vi "NI 9265 DOUBLE TASK.vi"(8 "error in":errorcluster, 11 "MODULE NAME":string="CDR_AO1") -> (0 "error out":errorcluster, 3 "task out":refnum<k21>)   [LabVIEW 2019]
uses:
  <vilib>/DAQmx/create/channels.llb/DAQmx Create Channel (AO-Current-Basic).vi
  <resource>/objmgr/daqmx.rc
panel:
  out "error out 2":errorcluster
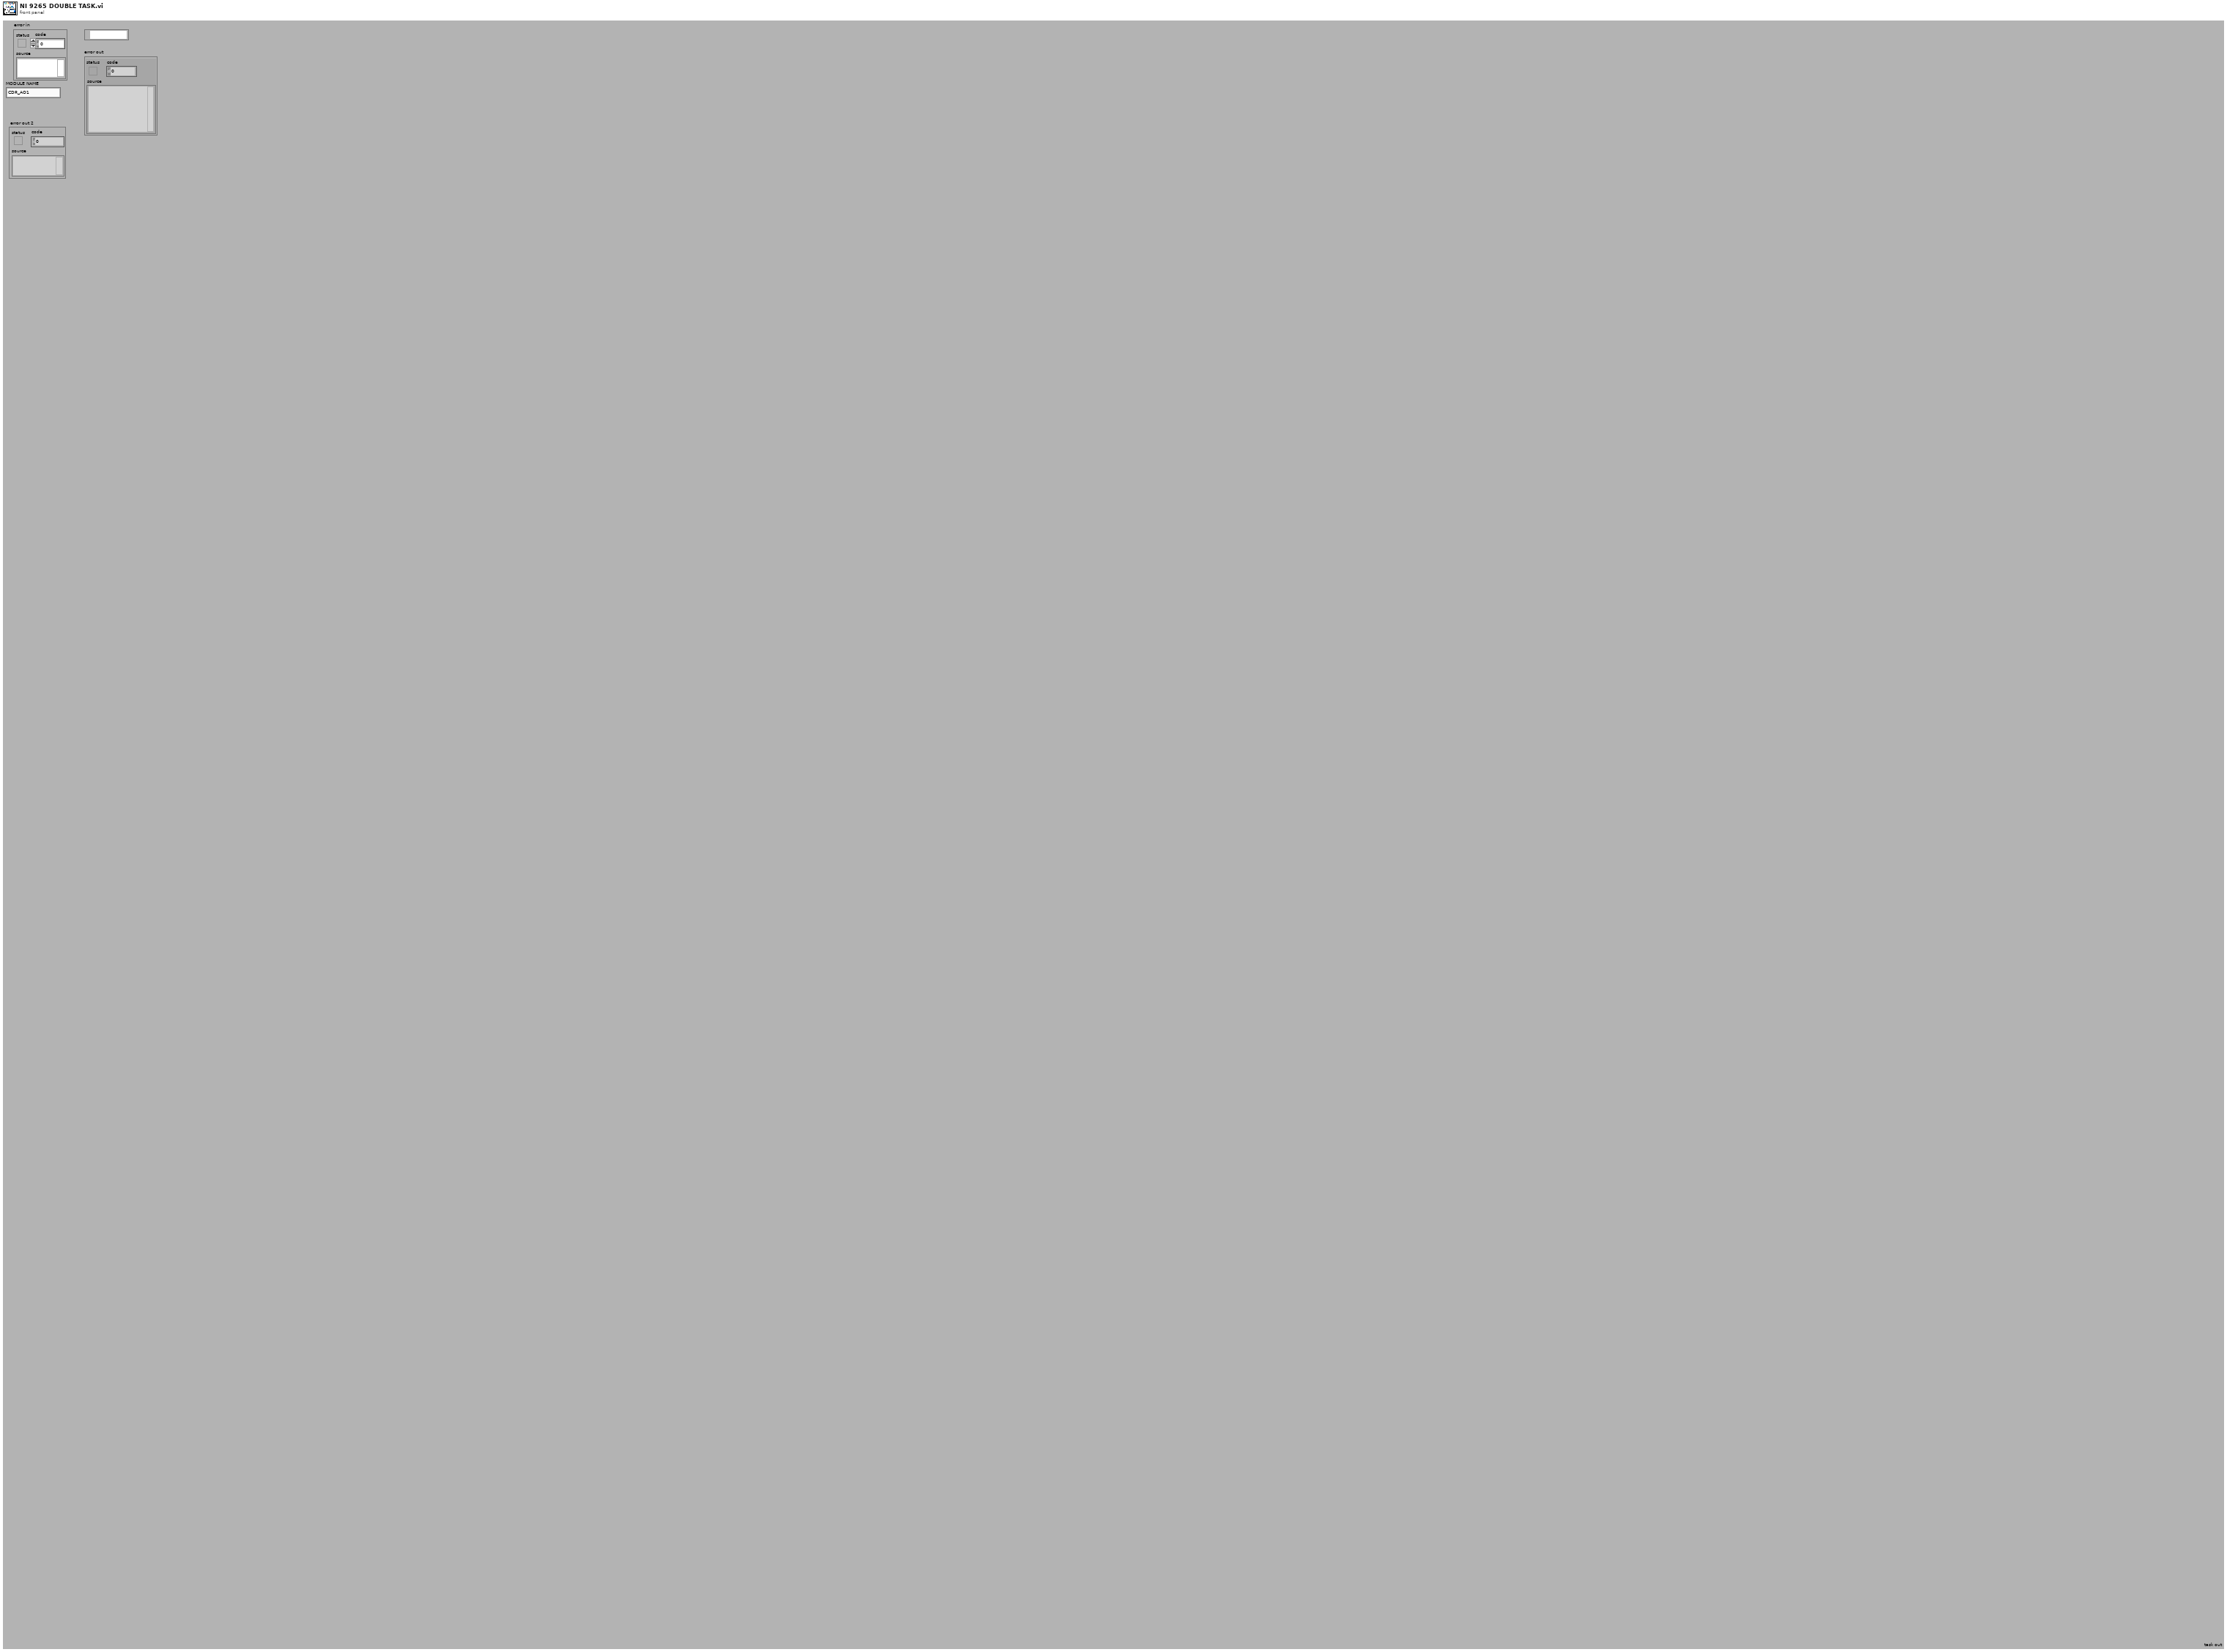
[diagram p1: front panel]
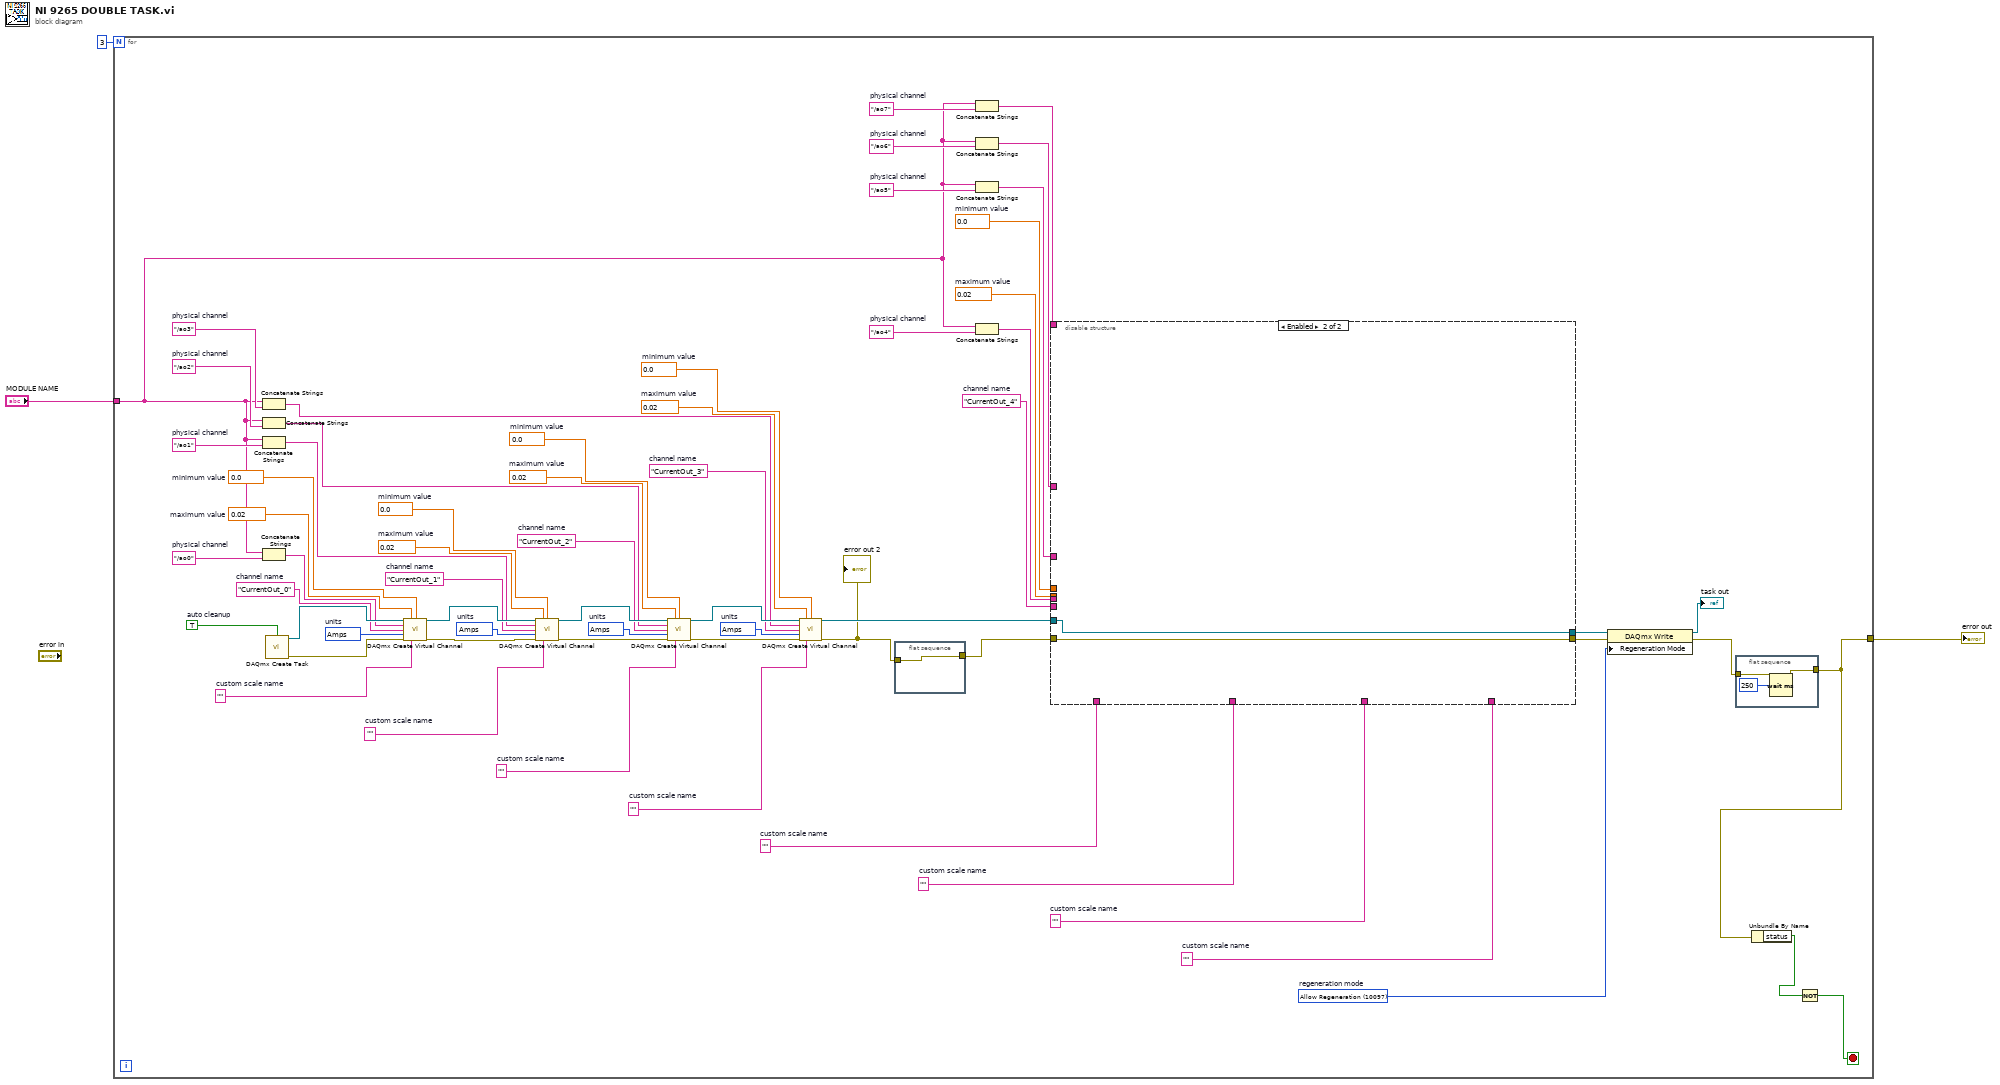
[diagram p0: block diagram]
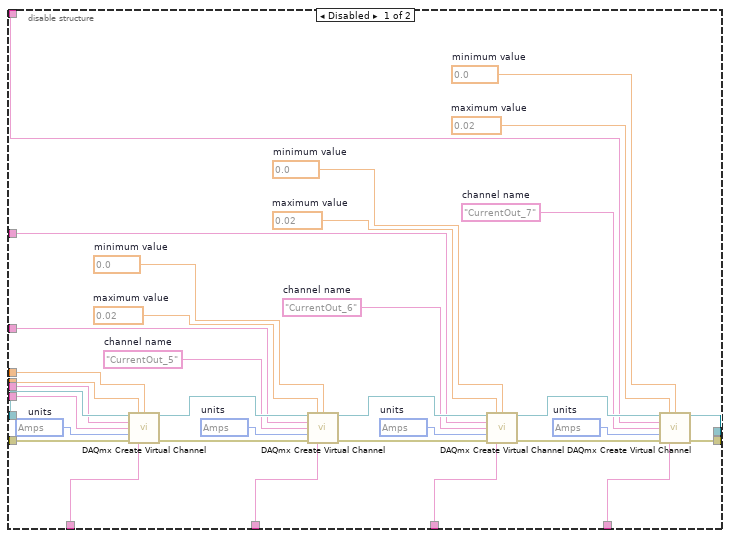
[diagram p2: hidden frame]
diagram:
  n1 = for {
    N: 3 -> [_]
    tunnel: "MODULE NAME" -> [w5]
    tunnel: [w8] -> w1
    stop <- w6 stop-if-true
    w13 = "/ao7"  # physical channel
    w15 = "/ao6"  # physical channel
    w17 = "/ao5"  # physical channel
    w20 = "CurrentOut_4"  # channel name
    w21 = 0.0  # minimum value
    w22 = 0.02  # maximum value
    w19 = "/ao4"  # physical channel
    w34 = 10097 items=["Allow Regeneration"=10097, "Do Not Allow Regeneration"=10158]  # regeneration mode
    w35 = ""  # custom scale name
    w36 = ""  # custom scale name
    w37 = ""  # custom scale name
    w38 = ""  # custom scale name
    w40 = 10342 items=["Amps"=10342, "From Custom Scale"=10065]  # units
    w41 = "CurrentOut_3"  # channel name
    w42 = ""  # custom scale name
    w43 = 0.0  # minimum value
    w44 = 0.02  # maximum value
    w25 = "/ao3"  # physical channel
    w46 = 10342 items=["Amps"=10342, "From Custom Scale"=10065]  # units
    w47 = "CurrentOut_2"  # channel name
    w49 = ""  # custom scale name
    w50 = 0.0  # minimum value
    w51 = 0.02  # maximum value
    w27 = "/ao2"  # physical channel
    w53 = 10342 items=["Amps"=10342, "From Custom Scale"=10065]  # units
    w54 = "CurrentOut_1"  # channel name
    w56 = ""  # custom scale name
    w57 = 0.0  # minimum value
    w58 = 0.02  # maximum value
    w28 = "/ao1"  # physical channel
    w60 = 10342 items=["Amps"=10342, "From Custom Scale"=10065]  # units
    w61 = "CurrentOut_0"  # channel name
    w62 = ""  # custom scale name
    w63 = 0.0  # minimum value
    w64 = 0.02  # maximum value
    w30 = "/ao0"  # physical channel
    w66 = TRUE  # auto cleanup
    n2 = Concatenate Strings(w5, w25) -> (w24:string)
    n3 = Concatenate Strings(w5, w27) -> (w26:string)
    n4 = Concatenate Strings(w5, w28) -> (w23:string)
    n5 = Concatenate Strings(w5, w30) -> (w29:string)
    n6 = call <vilib>:"DAQmx Create Task.vi"("auto cleanup"=w66) -> ("task out"=w65:refnum<k21>, "error out"=w67:errorcluster)  [unwired: 13 in]
    n7 = call-poly <vilib>:"DAQmx Create Virtual Channel.vi"("task in"=w65, "maximum value"=w64, "minimum value"=w63, "physical channels"=w29, "name to assign"=w61, "units"=w60, "error in"=w67, "custom scale name"=w62) -> ("task out"=w59:refnum<k21>, "error out"=w4:errorcluster)  [unwired: 6 in]
    n8 = call-poly <vilib>:"DAQmx Create Virtual Channel.vi"("task in"=w59, "maximum value"=w58, "minimum value"=w57, "physical channels"=w23, "name to assign"=w54, "units"=w53, "error in"=w4, "custom scale name"=w56) -> ("task out"=w52:refnum<k21>, "error out"=w55:errorcluster)  [unwired: 6 in]
    n9 = call-poly <vilib>:"DAQmx Create Virtual Channel.vi"("task in"=w52, "maximum value"=w51, "minimum value"=w50, "physical channels"=w26, "name to assign"=w47, "units"=w46, "error in"=w55, "custom scale name"=w49) -> ("task out"=w45:refnum<k21>, "error out"=w48:errorcluster)  [unwired: 6 in]
    n10 = call-poly <vilib>:"DAQmx Create Virtual Channel.vi"("task in"=w45, "maximum value"=w44, "minimum value"=w43, "physical channels"=w24, "name to assign"=w41, "units"=w40, "error in"=w48, "custom scale name"=w42) -> ("task out"=w39:refnum<k21>, "error out"=w10:errorcluster)  [unwired: 6 in]
    "error out 2" <- w10
    n11 = flat-sequence {
      tunnel: [w104] -> w9
      tunnel: w10 -> [w104]
      frame #0 {
      }
    }
    n12 = Concatenate Strings(w5, w13) -> (w12:string)
    n13 = Concatenate Strings(w5, w15) -> (w14:string)
    n14 = Concatenate Strings(w5, w17) -> (w16:string)
    n15 = Concatenate Strings(w5, w19) -> (w18:string)
    n16 = disable-structure shown="Enabled" {
      disable-tunnel: w39 -> [w101 w103]
      disable-tunnel: w38 -> [w100 _]
      disable-tunnel: w37 -> [w99 _]
      disable-tunnel: w36 -> [w98 _]
      disable-tunnel: w35 -> [w97 _]
      disable-tunnel: [w96 w103] -> w32
      disable-tunnel: [w95 w102] -> w31
      disable-tunnel: w22 -> [w94 _]
      disable-tunnel: w21 -> [w93 _]
      disable-tunnel: w20 -> [w91 _]
      disable-tunnel: w18 -> [w72 _]
      disable-tunnel: w16 -> [w71 _]
      disable-tunnel: w14 -> [w70 _]
      disable-tunnel: w12 -> [w69 _]
      disable-tunnel: w9 -> [w68 w102]
      frame Disabled {
        w73 = 10342 items=["Amps"=10342, "From Custom Scale"=10065]  # units
        w74 = "CurrentOut_7"  # channel name
        w75 = 0.0  # minimum value
        w76 = 0.02  # maximum value
        w78 = 10342 items=["Amps"=10342, "From Custom Scale"=10065]  # units
        w79 = "CurrentOut_6"  # channel name
        w81 = 0.0  # minimum value
        w82 = 0.02  # maximum value
        w84 = 10342 items=["Amps"=10342, "From Custom Scale"=10065]  # units
        w85 = "CurrentOut_5"  # channel name
        w87 = 0.0  # minimum value
        w88 = 0.02  # maximum value
        w90 = 10342 items=["Amps"=10342, "From Custom Scale"=10065]  # units
        n17 = call-poly <vilib>:"DAQmx Create Virtual Channel.vi"("task in"=w101, "maximum value"=w94, "minimum value"=w93, "physical channels"=w72, "name to assign"=w91, "units"=w90, "error in"=w68, "custom scale name"=w100) -> ("task out"=w89:refnum<k21>, "error out"=w92:errorcluster)  [unwired: 6 in]
        n18 = call-poly <vilib>:"DAQmx Create Virtual Channel.vi"("task in"=w89, "maximum value"=w88, "minimum value"=w87, "physical channels"=w71, "name to assign"=w85, "units"=w84, "error in"=w92, "custom scale name"=w99) -> ("task out"=w83:refnum<k21>, "error out"=w86:errorcluster)  [unwired: 6 in]
        n19 = call-poly <vilib>:"DAQmx Create Virtual Channel.vi"("task in"=w83, "maximum value"=w82, "minimum value"=w81, "physical channels"=w70, "name to assign"=w79, "units"=w78, "error in"=w86, "custom scale name"=w98) -> ("task out"=w77:refnum<k21>, "error out"=w80:errorcluster)  [unwired: 6 in]
        n20 = call-poly <vilib>:"DAQmx Create Virtual Channel.vi"("task in"=w77, "maximum value"=w76, "minimum value"=w75, "physical channels"=w69, "name to assign"=w74, "units"=w73, "error in"=w80, "custom scale name"=w97) -> ("task out"=w96:refnum<k21>, "error out"=w95:errorcluster)  [unwired: 6 in]
      }
      frame Enabled {
      }
    }
    n21 = property class="DAQmx Write"(reference=w32, error in=w31, "Regeneration Mode"=w34) -> (reference out=→"task out":refnum<k21>, error out=w11:errorcluster)
    n22 = flat-sequence {
      tunnel: [w105] -> w8
      tunnel: w11 -> [w105]
      frame #0 {
        n23 = Wait (ms)(milliseconds to wait=u32 250) -> ()  [unwired: 1 out]
      }
    }
    n24 = Unbundle By Name(w8) -> ("status"=w7:bool)
    n25 = Not(x=w7) -> (.not. x?=w6:bool)
  }
  "error out" <- w1
